vi "2D String Array_DeleteEmptyCells.vi"(2 "2D String Array.IN":string[][](array[string])=array16488x2[32976 elements]) -> (6 "2D String Array.OUT":string[][](array[string]))   [LabVIEW 2024]
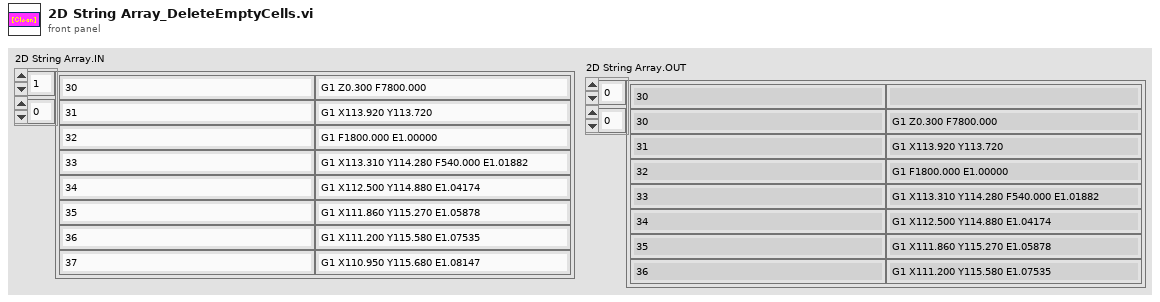
[diagram p1: front panel]
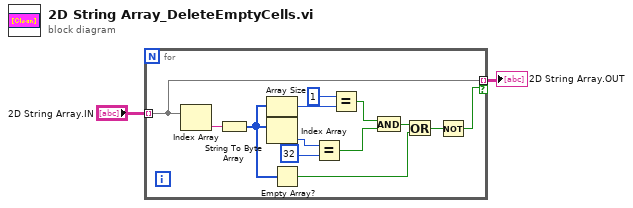
[diagram p0: block diagram]
diagram:
  n1 = for {
    tunnel: "2D String Array.IN" -> [w15] mode=indexing
    tunnel: [w15] -> w2 mode=indexing if=w3
    n2 = Index Array(array=w15) -> (element=w14:string)  [unwired: 1 in]
    n3 = String To Byte Array(string=w14) -> (unsigned byte array=w11:u8[])
    n4 = Array Size(array=w11) -> (size(s)=w10:i32)
    n5 = Index Array(array=w11) -> (element=w13:u8)  [unwired: 1 in]
    n6 = Empty Array?(array=w11) -> (empty?=w5:bool)
    n7 = Equal?(x=w13, y=u8 32) -> (x = y?=w7:bool)
    n8 = Equal?(x=1, y=w10) -> (x = y?=w8:bool)
    n9 = And(x=w8, y=w7) -> (x .and. y?=w6:bool)
    n10 = Or(x=w6, y=w5) -> (x .or. y?=w4:bool)
    n11 = Not(x=w4) -> (.not. x?=w3:bool)
  }
  "2D String Array.OUT" <- w2
